vi "Vision Tracking.vi"(11 "Ideal Target Height (in)":dbl) -> (2 "Distance (ft)":dbl, 3 "X-Value of Target":dbl)   [LabVIEW 2016]
uses:
  <vilib>/Rock Robotics/WPI/Camera/WPI_CameraSettings Read MJPG.ctl
  <vilib>/Rock Robotics/WPI/Camera/WPI_CameraImageSize.ctl
  Vision Support Code/Camera Types.ctl
  <vilib>/Rock Robotics/WPI/Camera/WPI_CameraExposure Values.ctl
  <vilib>/Rock Robotics/WPI/Camera/WPI_CameraWhite Balance Values.ctl
  <vilib>/vision/NI_Vision_Development_Module.lvlib
panel:
  in  "Line Border":cluster{"Top":dbl, "Bottom":dbl}={"Top"=6.0, "Bottom"=1.0}
  in  "Use Calibration":bool=TRUE
  out "Instructions:":string="Use Source to load image files from a directory, or use a USB or IP camera connected to your laptop. Use Camera Settings 1 and 2 to achieve a dark image with bright and colorful stripes.\nLED Color can encoded as HSL or related color modes. Calibrate to the same color as the strips being reflected to the camera.\nClick and draw a line in Original Image to auto-calibrate the LED Color. You may want to widen and tweak Sat and Val by hand.\nThe Annotate button affects drawing a rectangle around the stripes and labeling it with a distance in ft. Distance relies on knowing the Camera Type and lens calibration (it looks up the lens view angle).\n\nAdjust Score Cutoff to make the code more or less picky. If the color is not very unique, you may need to increase the number of particles considered. The diagram uses a Size Limit to ignore colored things that are too small. You may need to adjust it if you are targetting from far away.\n\nResults give you the distance to the target, the center and box in a normalized (-1 to 1) and pixel coordinates.\n\nBe sure to read about setting camera exposure and brightness to help simplify your image and acquire color saturated images.\n\nThere are lots of comments on the diagram to explain the code."
  in  "Color Mode":u16(ring)=3 items=["RGB", "HSL", "HSV", "HSI"]
  in  "Particles":dbl=5.0
  in  "Score Cutoff %":dbl=70.0
  in  "Std Devs for Calibration":cluster{"H":dbl, "S":dbl, "V":dbl}={"H"=4.0, "S"=6.0, "V"=6.0}
  in  "Camera Type":T1=enum."MS HD3000 square"
  in  "image files":string[](array[string])
  out "Results":T2 {"Score" format="%#_3g"; "Pixels"."Rectangle"."Numeric 5" format="%#_3g"; "Pixels"."Rectangle"."Numeric 3" format="%#_3g"; "Pixels"."Rectangle"."Numeric 2" format="%#_3g"; "Pixels"."Rectangle"."Numeric" format="%#_3g"; "Normalized"."Rectangle"."Numeric 5" format="%#_2g"; "Normalized"."Rectangle"."Numeric 3" format="%#_2g"; "Normalized"."Rectangle"."Numeric 2" format="%#_2g"; "Normalized"."Rectangle"."Numeric" format="%#_2g"; "Normalized"."Center"."?" format="%#_3g"; "Normalized"."Center"."?" format="%#_3g"; "Distance (ft)" format="%#_3g"}
  in  "Source":enum32{"Files", "Camera"}(tab)
  in  "Images":i32(listbox)
  in  "Folder Location":path=path "C:/Program Files (x86)/National Instruments/LabVIEW 2016/examples/FRC/roboRIO/Vision/2017 Vision Example/Sample Images/LED Boiler"
  in  "Camera Settings":T3={"fps"=20, "compression"=30, "Image Size"=enum."320x240", "Config Shown"=FALSE}
  in  "Camera Address":string="USB 1"
  in  "Camera Settings 2":T7={"Exposure"=enum."Auto", "Exposure (%)"=50.0, "Brightness"=50, "White Balance"=enum."Auto", "Color Temp (K)"=0.0} {"Brightness" min=0 max=100}
  in  "Annotate":bool=TRUE
  out "Qualified Particles":i32
  in  "LED Color":T8={"Hue"={107.81818389892578, 139.81818389892578}, "Sat"={176.07142857142858, 255.0}, "Val"={40.53571428571429, 255.0}} {"Hue" scale=0.0..255.0 scale format="%#_3g"}
  out "Mask":T9(plugin-control)
  out "Original Image":T9(plugin-control)
  # "Legend:\n    Rectangle\n       Green - Good target, distance ft\n       Red - Bad target\n    Orange Text - Score in %"
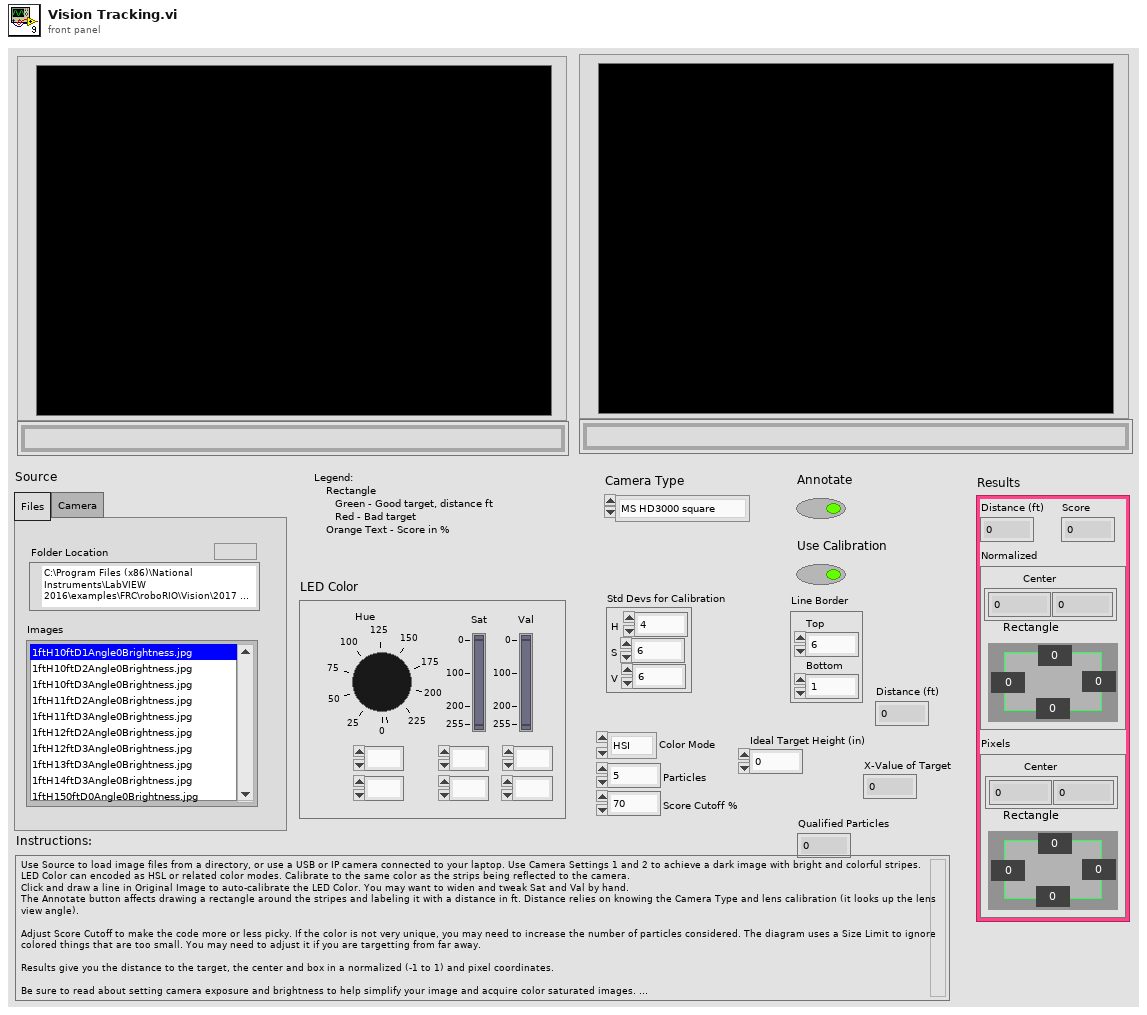
[diagram p1: front panel]
types:
  T1 = typedef "Camera Types.ctl" = enum16{"206", "1011", "1013", "MS HD3000 square", "MS HD3000 640x480"}
  T2 = cluster{"Distance (ft)":dbl, "Score":dbl, "Normalized":cluster{"Center":cluster{dbl, dbl}, "Rectangle":cluster{"Numeric":dbl, "Numeric 2":dbl, "Numeric 3":dbl, "Numeric 5":dbl}}, "Pixels":cluster{"Center":cluster{dbl, dbl}, "Rectangle":cluster{"Numeric":dbl, "Numeric 2":dbl, "Numeric 3":dbl, "Numeric 5":dbl}}}
  T3 = typedef "WPI_CameraSettings Read MJPG.ctl" = cluster{"fps":i32, "compression":i32, "Image Size":T4, "Config Shown":bool}
  T4 = typedef "WPI_CameraImageSize.ctl" = enum16{"640x480", "320x240", "160x120", "Custom"}
  T5 = typedef "WPI_CameraExposure Values.ctl" = enum16{"Auto", "Flicker-free 50 Hz", "Flicker-free 60 Hz", "Hold current", "Custom"}
  T6 = typedef "WPI_CameraWhite Balance Values.ctl" = enum16{"Auto", "Fixed indoor", "Fixed outdoor 1", "Fixed outdoor 2", "Fixed fluorescent 1", "Fixed fluorescent 2", "Hold current", "Custom"}
  T7 = cluster{"Exposure":T5, "Exposure (%)":dbl, "Brightness":i32, "White Balance":T6, "Color Temp (K)":dbl}
  T8 = cluster{"Hue":cluster{dbl, dbl}, "Sat":cluster{dbl, dbl}, "Val":cluster{dbl, dbl}}
  T9 = typedef "IMAQ Image.ctl" = refnum<image>
  T10 = typedef "Image Type" = u32
  T11 = typedef "Particle Parameters" = i32
  T12 = cluster{cluster{dbl, dbl}, cluster{dbl, dbl}, cluster{dbl, dbl}}
  T13 = cluster{"Left":dbl, "Top":dbl, "Right":dbl, "Bottom":dbl}
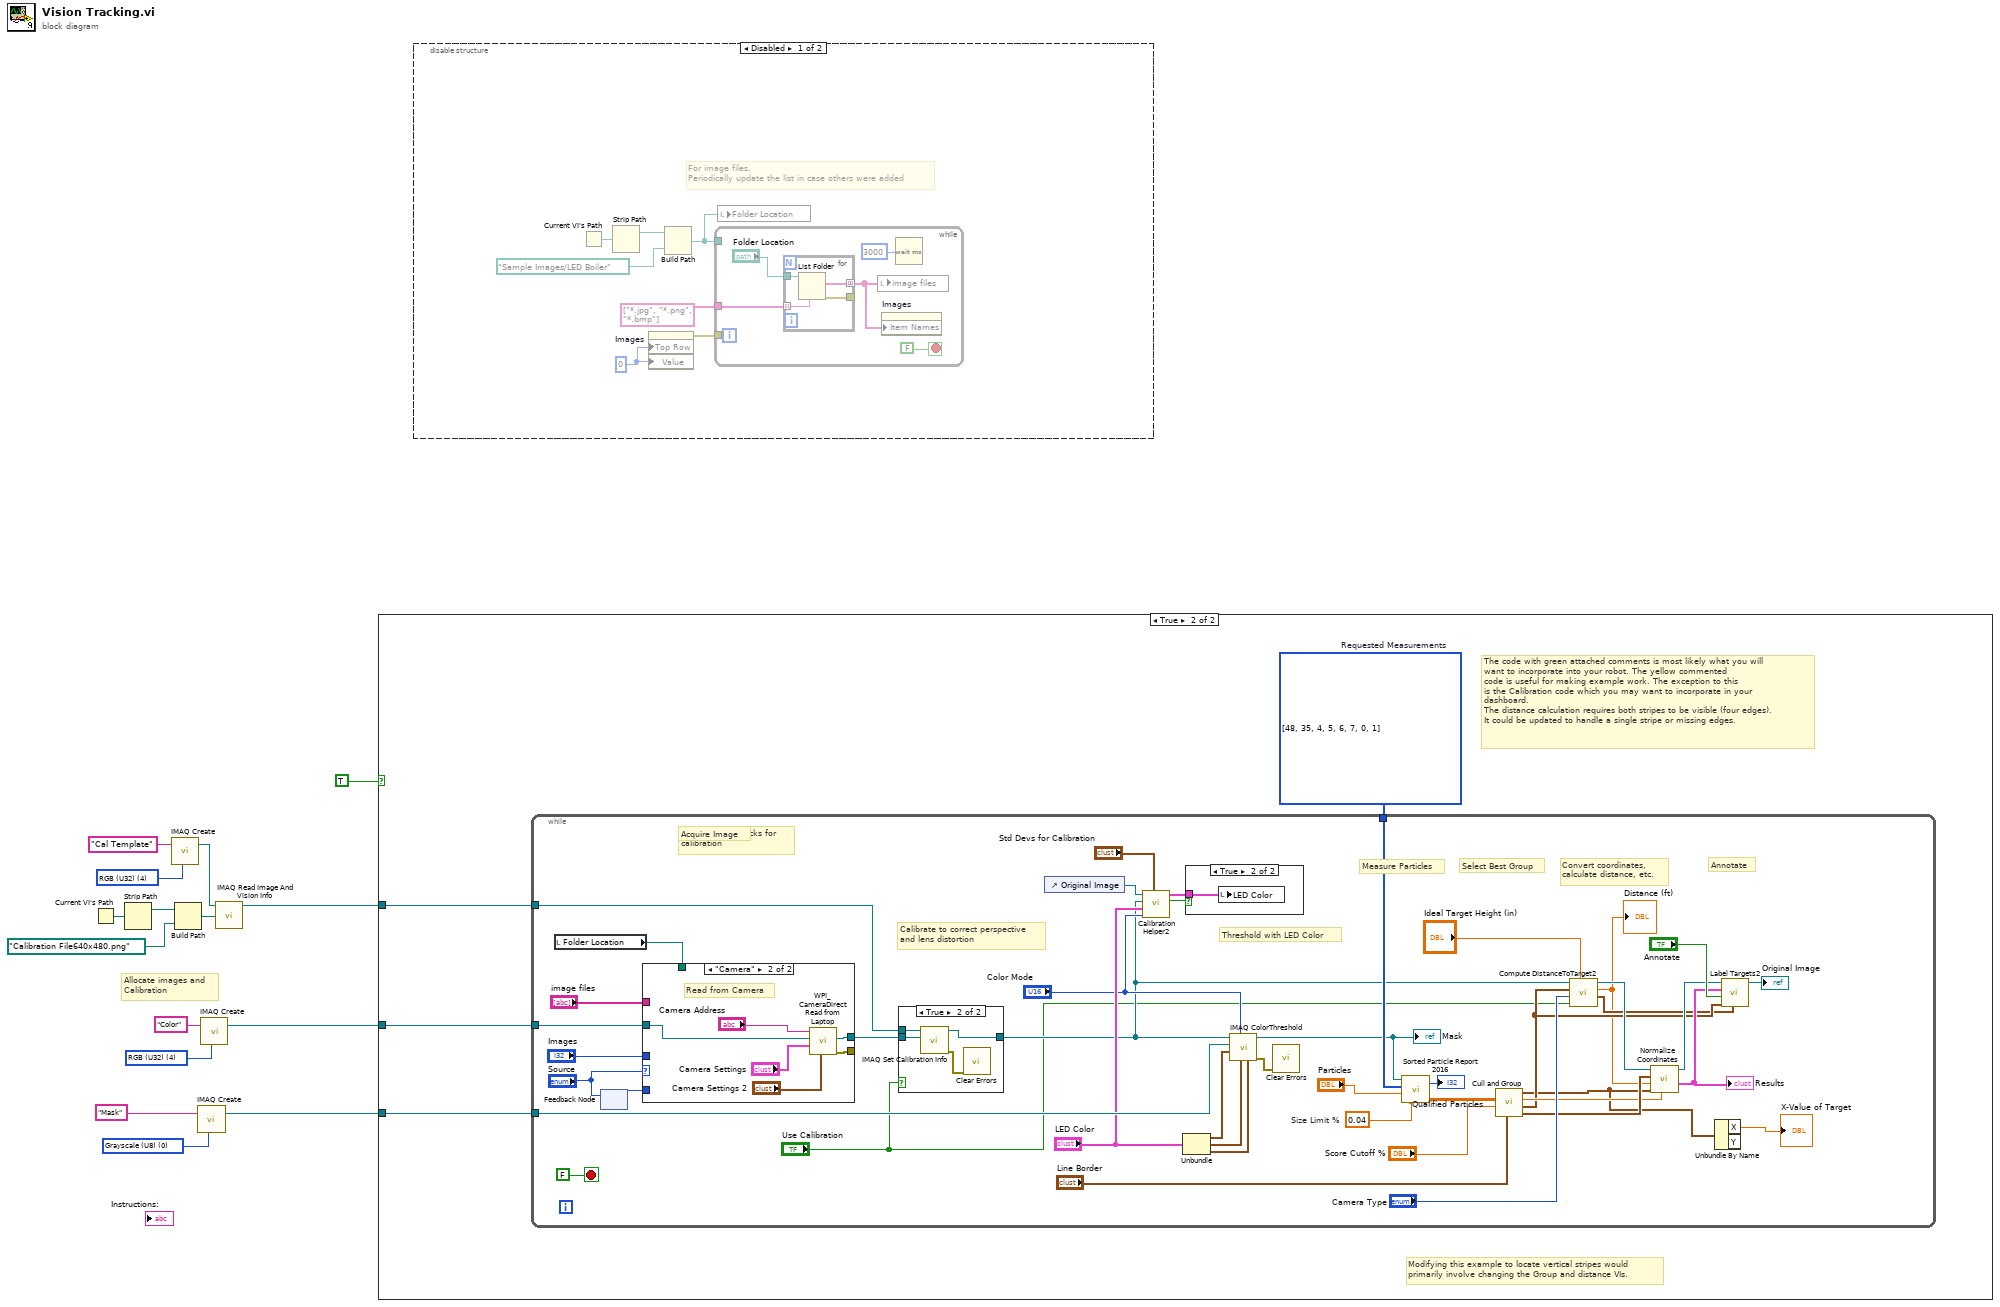
[diagram p0: block diagram]
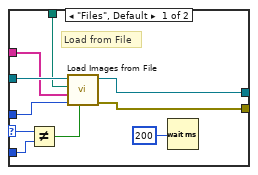
[diagram p5: hidden frame]
diagram:
  w9 = T10 4 items=["Grayscale (U8)", "Grayscale (I16)", "Grayscale (SGL)", "Complex (CSG)", "RGB (U32)", "HSL (U32)", "RGB (U64)", "Grayscale (U16)"] ("Image Type")
  w13 = T10 0 items=["Grayscale (U8)", "Grayscale (I16)", "Grayscale (SGL)", "Complex (CSG)", "RGB (U32)", "HSL (U32)", "RGB (U64)", "Grayscale (U16)"] ("Image Type")
  w14 = T10 4 items=["Grayscale (U8)", "Grayscale (I16)", "Grayscale (SGL)", "Complex (CSG)", "RGB (U32)", "HSL (U32)", "RGB (U64)", "Grayscale (U16)"] ("Image Type")
  # "Allocate images and\nCalibration"
  n1 = Current VI's Path() -> (path=w5:path)
  n2 = Strip Path(path=w5) -> (stripped path=w2:path)  [unwired: 1 out]
  n3 = call "IMAQ Create"("Image Name"="Cal Template", "Image Type"=w9) -> ("New Image"=w7:T9)  [unwired: 2 in, 2 out]
  n4 = Build Path(base path=w2, name or relative path=path "Calibration File640x480.png" ("Folder Location")) -> (appended path=w4:path)
  n5 = call "IMAQ Create"("Image Name"="Mask", "Image Type"=w13) -> ("New Image"=w11:T9)  [unwired: 2 in, 2 out]
  n6 = call "IMAQ Create"("Image Name"="Color", "Image Type"=w14) -> ("New Image"=w10:T9)  [unwired: 2 in, 2 out]
  n7 = call "IMAQ Read Image And Vision Info"("File Path"=w4, "Image"=w7) -> ("Image Out"=w6:T9)  [unwired: 7 in, 2 out]
  n8 = case shown="True" TRUE {
    tunnel: w11 -> [_ w19]
    tunnel: w10 -> [_ w17]
    tunnel: w6 -> [_ w16]
    frame False {
    }
    frame True {
      w18 = T11[] [48, 35, 4, 5, 6, 7, 0, 1] items=["Center of Mass X", "Center of Mass Y", "First Pixel X", "First Pixel Y", "Bounding Rect Left", "Bounding Rect Top", "Bounding Rect Right", "Bounding Rect Bottom", "Max Feret Diameter Start X", "Max Feret Diameter Start Y", "Max Feret Diameter End X", "Max Feret Diameter End Y", "Max Horiz. Segment Length Left", "Max Horiz. Segment Length Right", "Max Horiz. Segment Length Row", "-", "Bounding Rect Width", "Bounding Rect Height", "Bounding Rect Diagonal", "Perimeter", "Convex Hull Perimeter", "Holes' Perimeter", "Max Feret Diameter", "Equivalent Ellipse Major Axis", "Equivalent Ellipse Minor Axis", "Equivalent Ellipse Minor Axis (Feret)", "Equivalent Rect Long Side", "Equivalent Rect Short Side", "Equivalent Rect Diagonal", "Equivalent Rect Short Side (Feret)", "Average Horiz. Segment Length", "Average Vert. Segment Length", "Hydraulic Radius", "Waddel Disk Diameter", "-", "Area", "Holes' Area", "Particle & Holes' Area", "Convex Hull Area", "Image Area", "-", "Number of Holes", "Number of Horiz. Segments", "Number of Vert. Segments", "-", "Orientation", "Max Feret Diameter Orientation", "-", "% Area/Image Area", "% Area/(Particle & Holes' Area)", "Ratio of Equivalent Ellipse Axes", "Ratio of Equivalent Rect Sides", "-", "Elongation Factor", "Compactness Factor", "Heywood Circularity Factor", "Type Factor", "-", "Sum X", "Sum Y", "Sum XX", "Sum XY", "Sum YY", "Sum XXX", "Sum XXY", "Sum XYY", "Sum YYY", "-", "Moment of Inertia XX", "Moment of Inertia XY", "Moment of Inertia YY", "Moment of Inertia XXX", "Moment of Inertia XXY", "Moment of Inertia XYY", "Moment of Inertia YYY", "Norm. Moment of Inertia XX", "Norm. Moment of Inertia XY", "Norm. Moment of Inertia YY", "Norm. Moment of Inertia XXX", "Norm. Moment of Inertia XXY", "Norm. Moment of Inertia XYY", "Norm. Moment of Inertia YYY", "Hu Moment 1", "Hu Moment 2", "Hu Moment 3", "Hu Moment 4", "Hu Moment 5", "Hu Moment 6", "Hu Moment 7"]  # Requested Measurements
      # "Modifying this example to locate vertical stripes would\nprimarily involve changing the Group and distance VIs."
      # "The code with green attached comments is most likely what you will\nwant to incorporate into your robot. The yellow commented\ncode is useful for making example work. The exception to this\nis the Calibration code which you may want to incorporate in your\ndashboard.\nThe distance calculation requires both stripes to be visible (four edges).\nIt could be updated to handle a single stripe or missing edges."
      n9 = while {
        tunnel: w17 -> [w62]
        tunnel: w19 -> [w60]
        tunnel: w18 -> [w56]
        tunnel: w16 -> [w26]
        stop <- FALSE stop-if-true
        w54 = 0.04  # Size Limit %
        # "Calibrate to correct perspective\nand lens distortion"
        # "Handle Mouse clicks for\ncalibration"
        # "Measure Particles"
        # "Convert coordinates,\ncalculate distance, etc."
        # "Annotate"
        # "Select Best Group"
        # "Threshold with LED Color"
        # "Acquire Image"
        n10 = local read "Folder Location"() -> (w44:path)
        n11 = feedback-in #1("Source") -> ()
        n12 = feedback #1() -> (w42:enum32{"Files", "Camera"})  [unwired: 1 in]
        n13 = case shown="\"Camera\"" "Source" {
          selector: "Source" -> [w72 _]
          tunnel: [w78 w85] -> _
          tunnel: [w79 w84] -> w27
          tunnel: w62 -> [w77 w83]
          tunnel: "image files" -> [w74 _]
          tunnel: "Images" -> [w76 _]
          tunnel: w44 -> [w75 _]
          tunnel: w42 -> [w71 _]
          frame "Files", Default {
            # "Load from File"
            n14 = Not Equal?(x=w72, y=w71) -> (x != y?=w70:bool)
            n15 = call "Load Images from File.vi"("Force Load"=w70, "Images"=w76, "image files"=w74, "Folder Location"=w75, "Refnum in"=w77) -> ("error out"=w78:errorcluster, "Refnum out"=w79:T9)  [unwired: 5 in]
            n16 = Wait (ms)(milliseconds to wait=u32 200 ("delay (ms)")) -> ()  [unwired: 1 out]
          }
          frame "Camera" {
            # "Read from Camera"
            n17 = call <vilib>:"WPI_CameraDirect Read from Laptop.vi"("Camera Settings 2"="Camera Settings 2", "Camera Settings"="Camera Settings", "Image"=w83, "address"="Camera Address") -> ("error out"=w85:errorcluster, "Image Out"=w84:T9)  [unwired: 6 in]
          }
        }
        n18 = case shown="True" "Use Calibration" {
          tunnel: [w64 w68] -> w28
          tunnel: w27 -> [w64 w67]
          tunnel: w26 -> [_ w66]
          frame False {
          }
          frame True {
            n19 = call "IMAQ Set Calibration Info"("Image Dst"=w67, "Image Src"=w66) -> ("error out"=w65:errorcluster, "Calibrated Image"=w68:T9)  [unwired: 8 in]
            n20 = call <vilib>:"Clear Errors.vi"("error in (no error)"=w65) -> ()  [unwired: 5 in, 2 out]
          }
        }
        n21 = control-ref of="Original Image"() -> (w49:refnum<vi>)
        n22 = call "Calibration Helper2.vi"("Std Devs"="Std Devs for Calibration", "Color Mode"="Color Mode", "Color Components"="LED Color", "Image"=w28, "Image Ctl Refnum"=w49) -> ("Changed"=w48:bool, "output color"=w47:T12)  [unwired: 5 in]
        n23 = Unbundle("LED Color") -> ("Hue"=w59:cluster{dbl, dbl}, "Sat"=w58:cluster{dbl, dbl}, "Val"=w57:cluster{dbl, dbl})
        n24 = case shown="True" w48 {
          tunnel: w47 -> [_ w69]
          frame False {
          }
          frame True {
            n25 = local write "LED Color"(w69) -> ()
          }
        }
        n26 = call "IMAQ ColorThreshold"("Blue or Luma or Val or Inten Range"=w57, "Green or Sat Range"=w58, "Color Mode"="Color Mode", "Red or Hue Range"=w59, "Image Dst"=w60, "Image Src"=w28) -> ("error out"=w50:errorcluster, "Image Dst Out"=w39:T9)  [unwired: 4 in]
        "Mask" <- w39
        n27 = call <vilib>:"Clear Errors.vi"("error in (no error)"=w50) -> ()  [unwired: 5 in, 2 out]
        n28 = call "Sorted Particle Report 2016.vi"("Min Area Size %"=w54, "Particle Count Limit"="Particles", "Pixel Measurements"=w56, "Image in"=w39) -> ("Sorted Data"=w41:dbl[][], "Particles"=→"Qualified Particles":i32)
        n29 = call "Cull and Group.vi"("Line Border"="Line Border", "Score Cutoff"="Score Cutoff %", "Sorted Data"=w41) -> ("Rect"=w37:T13, "Line"=w30:T13, "Score"=w33:dbl, "Center"=w23:cluster{"X":dbl, "Y":dbl})  [unwired: 5 in]
        n30 = call "Compute DistanceToTarget2.vi"("Ideal Target Height (in)"="Ideal Target Height (in)", "Calibrated"="Use Calibration", "Camera Type"="Camera Type", "Line"=w30, "Image Src"=w28) -> ("Edges"=w29:cluster{"X":sgl, "Y":sgl}[], "Distance (ft)"=w20:dbl, "Image Dst Out"=w36:T9)  [unwired: 4 in]
        "Distance (ft)" <- w20
        n31 = call "Normalize Coordinates.vi"("Score"=w33, "Center"=w23, "Distance"=w20, "Bounding box"=w37, "Image in"=w36) -> ("Results"=w34:T2, "Image out"=w35:T9)  [unwired: 5 in]
        "Results" <- w34
        n32 = Unbundle By Name(w23) -> ("X"=→"X-Value of Target":dbl)  [unwired: 1 out]
        n33 = call "Label Targets2.vi"("Edges"=w29, "Line"=w30, "Annotate"="Annotate", "Results"=w34, "Image in"=w35) -> ("Image out"=→"Original Image":T9)  [unwired: 6 in]
      }
    }
  }
  n34 = disable-structure shown="Disabled" {
    frame Disabled {
      w87 = u32 0 ("milliseconds to wait")
      # "For image files.\nPeriodically update the list in case others were added"
      n35 = Current VI's Path() -> (path=w92:path)
      n36 = Strip Path(path=w92) -> (stripped path=w90:path)  [unwired: 1 out]
      n37 = property on="Images" class="LstBox (strict)"("Top Row"=w87, "Value"=w87) -> (error out=w88:errorcluster)  [unwired: 2 in, 1 out]
      n38 = Build Path(base path=w90, name or relative path=path "Sample Images/LED Boiler" ("Folder Location")) -> (appended path=w89:path)
      n39 = while {
        tunnel: w89 -> [_]
        tunnel: w88 -> [_]
        tunnel: string[] ["*.jpg", "*.png", "*.bmp"] -> [w94]
        stop <- FALSE stop-if-true
        n40 = for {
          tunnel: [w101] -> w96 mode=concatenating
          tunnel: "Folder Location" -> [w100]
          tunnel: [w99] -> _
          tunnel: w94 -> [w98] mode=indexing
          n41 = List Folder(path=w100, pattern=w98) -> (filenames=w101:string[], error out=w99:errorcluster)  [unwired: 2 in, 2 out]
        }
        n42 = local write "image files"(w96) -> ()
        n43 = property on="Images" class="LstBox (strict)"("Item Names"=w96) -> ()  [unwired: 2 in, 2 out]
        n44 = Wait (ms)(milliseconds to wait=u32 3000) -> ()  [unwired: 1 out]
      }
      n45 = local write "Folder Location"(w89) -> ()
    }
    frame Enabled {
    }
  }
